vi "Measure Resistance.vi"(8 "error in":errorcluster, 10 "range":dbl=20000.0 caption="Range (20k)" format="%.2f", 11 "instrument handle":refnum<k15>="IVI-KE2000") -> (0 "error out":errorcluster, 2 "Resistance":dbl[unit]=nan caption="Measurement" format="%.2f", 3 "instrument handle 2":refnum<k15> caption="instrument handle")   [LabVIEW 2010]
doc: "This function performs a 4-wire resistance measurement with a DMM."
panel:
  in  "trigger source (Imm)":i32(ring)=1 caption="trigger source (Immediate)" items=["Immediate"=1, "External"=2, "Software Trigger Function"=3, "PXI TRIG0 or VXI TTL0"=111, "PXI TRIG1 or VXI TTL1"=112, "PXI TRIG2 or VXI TTL2"=113, "PXI TRIG3 or VXI TTL3"=114, "PXI TRIG4 or VXI TTL4"=115, "PXI TRIG5 or VXI TTL5"=116, "PXI TRIG6 or VXI TTL6"=117, "PXI TRIG7 or VXI TTL7"=118, "ECL0"=119, "ECL1"=120, "PXI Star"=131, "RTSI 0"=140, "RTSI 1"=141, "RTSI 2"=142, "RTSI 3"=143, "RTSI 4"=144, "RTSI 5"=145, "RTSI 6"=146]
  in  "function (4-Wire)":i32(ring)=101 caption="measurement function (DC Volts)" items=["DC Volts"=1, "AC Volts"=2, "DC Current"=3, "AC Current"=4, "2 Wire Resistance"=5, "4 Wire Resistance"=101, "AC + DC Volts"=106, "AC + DC Current"=107, "Frequency"=104, "Period"=105, "Temperature"=108]
  in  "max time (ms)":i32=5000 caption="Max Time (ms)"
  in  "resolution":dbl=1e-05 caption="Resolution" format="%.5f"
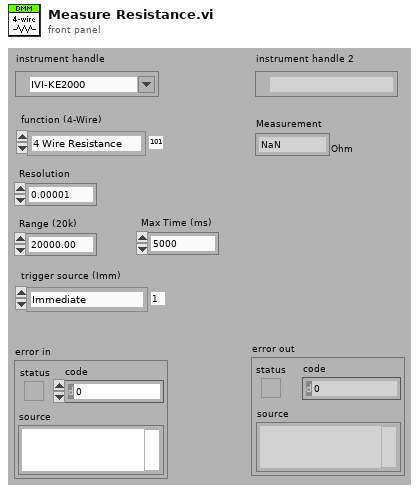
[diagram p1: front panel]
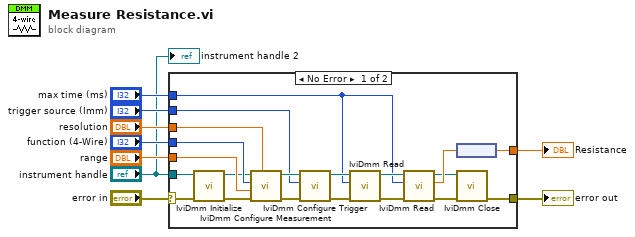
[diagram p0: block diagram]
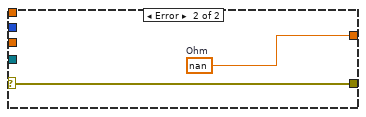
[diagram p2: hidden frame]
diagram:
  n1 = case shown="No Error" "error in" {
    selector: "error in" -> [w16 w31]
    tunnel: "resolution" -> [w29 _]
    tunnel: "range" -> [w28 _]
    tunnel: "trigger source (Imm)" -> [w17 _]
    tunnel: "max time (ms)" -> [w22 _]
    tunnel: [w20 w30] -> w6
    tunnel: [w12 w31] -> w4
    tunnel: "function (4-Wire)" -> [w19 _]
    tunnel: "instrument handle" -> [w14 _]
    frame No Error {
      n2 = call <vilib>:"IviDmm Initialize.vi"("error in (no error)"=w16, "logical name (\"SampleDmm\")"=w14) -> ("error out"=w15:errorcluster, "instrument handle out"=w10:refnum<k15>)  [unwired: 8 in]
      n3 = call <vilib>:"IviDmm Configure Measurement.vi"("absolute resolution (0.001)"=w29, "error in (no error)"=w15, "range (-1.0: Auto)"=w28, "measurement function (DC Volts)"=w19, "instrument handle"=w10) -> ("error out"=w27:errorcluster, "instrument handle out"=w18:refnum<k15>)  [unwired: 5 in]
      n4 = call <vilib>:"IviDmm Configure Trigger.vi"("error in (no error)"=w27, "trigger source (Immediate)"=w17, "instrument handle"=w18) -> ("error out"=w26:errorcluster, "instrument handle out"=w25:refnum<k15>)  [unwired: 7 in]
      n5 = call <vilib>:"IviDmm Read.vi"("error in (no error)"=w26, "maximum time (5000 ms)"=w22, "instrument handle"=w25) -> ("error out"=w24:errorcluster, "instrument handle out"=w23:refnum<k15>)  [unwired: 6 in, 1 out]
      n6 = call <vilib>:"IviDmm Read.vi"("error in (no error)"=w24, "maximum time (5000 ms)"=w22, "instrument handle"=w23) -> ("error out"=w13:errorcluster, "reading"=w21:dbl, "instrument handle out"=w11:refnum<k15>)  [unwired: 6 in]
      n7 = node(w21) -> (w20:dbl[unit])
      n8 = call <vilib>:"IviDmm Close.vi"("error in (no error)"=w13, "instrument handle"=w11) -> ("error out"=w12:errorcluster)  [unwired: 9 in]
    }
    frame Error {
      w30 = dbl[unit] nan  # Ohm
    }
  }
  "Resistance" <- w6
  "error out" <- w4
  "instrument handle 2" <- "instrument handle"
